vi "DSF.Shared.Configuration.Transfer.Compact Channels.vi"(11 "Channel Parameters":T2[](array[typedef]) {"Channel Ref" format="%016x"; "offset" format="%d bytes"}) -> (3 "Channel Blocks":T1[](array[typedef]) {"count" format="%d elements"; "Base Channel"."Channel Ref" format="%016x"; "Base Channel"."offset" format="%d bytes"})   [LabVIEW 2016, in "DSF.Shared.lvlib" / "DSF.Shared.Configuration.Transfer.lvclass"]
uses:
  DSF.Shared.Configuration.Transfer.lvclass
  Typedefs/DSF.Shared.Typedefs.Configuration.Transfer.Channel Parameters.ctl
  Typedefs/DSF.Shared.Typedefs.Data Type.ctl
  <vilib>/NI Veristand/Custom Device API/Custom Device Item Ref.ctl
  Typedefs/DSF.Shared.Typedefs.Configuration.Transfer.Channel Block.ctl
  DSF.Shared.lvlib
  <vilib>/NI Veristand/Custom Device API/Custom Device API.lvlib
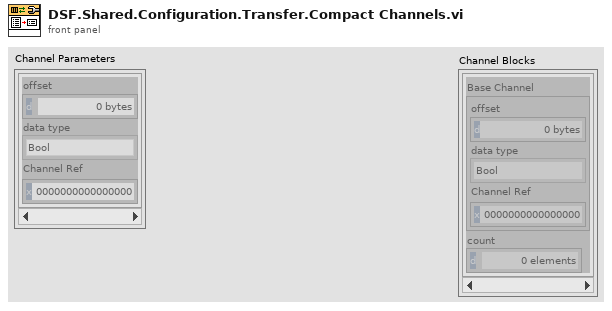
[diagram p1: front panel]
types:
  T1 = typedef "DSF.Shared.lvlib/DSF.Shared.Typedefs.Configuration.Transfer.Channel Block.ctl" = cluster{"Base Channel":T2, "count":u64}
  T2 = typedef "DSF.Shared.lvlib/DSF.Shared.Typedefs.Configuration.Transfer.Channel Parameters.ctl" = cluster{"offset":u64, "data type":T3, "Channel Ref":T4}
  T3 = typedef "DSF.Shared.lvlib/DSF.Shared.Typedefs.Data Type.ctl" = enum8{"Bool", "SGL", "DBL", "I8", "I16", "I32", "I64", "U8", "U16", "U32", "U64"}
  T4 = typedef "Custom Device API.lvlib/Custom Device Item Ref.ctl" = u64
  T5 = cluster{"offset":bool, "data type":bool, "Channel Ref":bool}
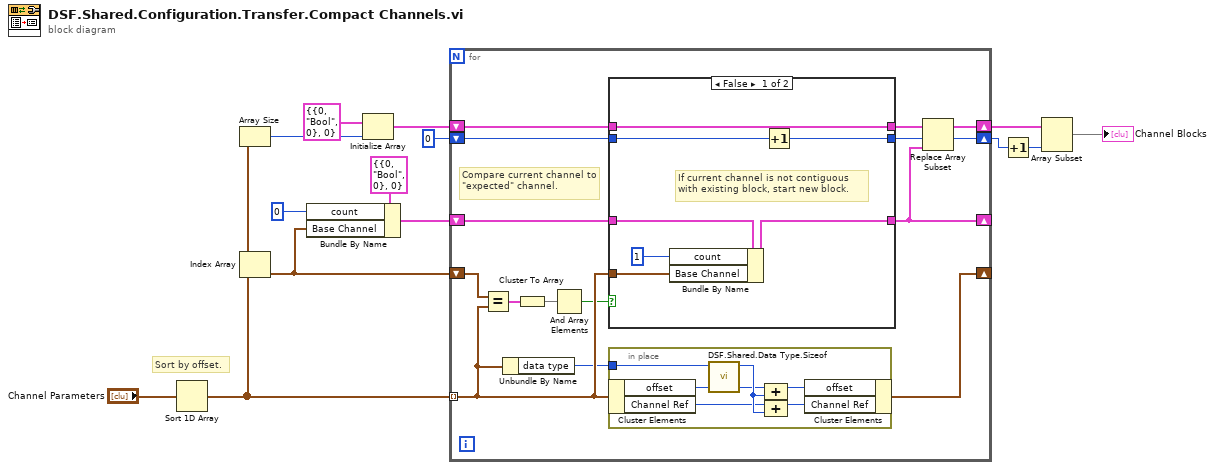
[diagram p0: block diagram]
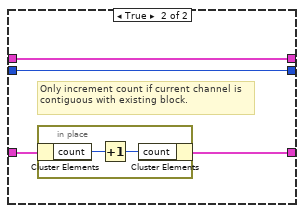
[diagram p2: hidden frame]
diagram:
  # "Sort by offset."
  n1 = Sort 1D Array(array="Channel Parameters") -> (sorted array=w6:T2[])
  n2 = Array Size(array=w6) -> (size(s)=w12:i32)
  n3 = Index Array(array=w6) -> (element=w4:T2)  [unwired: 1 in]
  n4 = Bundle By Name(cluster=T1 {"Base Channel"={"offset"=0, "data type"=enum."Bool", "Channel Ref"=0}, "count"=0} ("Channel Parameters"), "count"=u64 0, "Base Channel"=w4) -> (w3:T1)
  n5 = Initialize Array(T1 {"Base Channel"={"offset"=0, "data type"=enum."Bool", "Channel Ref"=0}, "count"=0} ("Channel Parameters"), w12) -> (w11:T1[])
  n6 = for {
    tunnel: w6 -> [w28] mode=indexing
    shift-right: [w17] -> _
    shift-left: w4 -> [w25]
    shift-right: [w20] -> w9
    shift-left: w11 -> [w23]
    shift-right: [w19] -> w8
    shift-left: 0 ("size(s)") -> [w22]
    shift-right: [w18] -> _
    shift-left: w3 -> [w24]
    # "Compare current channel to \"expected\" channel."
    n7 = Equal?(x=w25, y=w28) -> (x = y?=w27:T5)
    n8 = Unbundle By Name(w28) -> ("data type"=w16:T3)
    n9 = Cluster To Array(cluster=w27) -> (array=w26:bool[])
    n10 = And Array Elements(Boolean array=w26) -> (logical AND=w15:bool)
    n11 = case shown="False" w15 {
      tunnel: w24 -> [w39 w45]
      tunnel: [w38 w44] -> w18
      tunnel: w23 -> [w40 w43]
      tunnel: w22 -> [w41 w42]
      tunnel: [w37 w42] -> w19
      tunnel: [w40 w43] -> w21
      tunnel: w28 -> [w35 _]
      frame False {
        # "If current channel is not contiguous with existing block, start new block."
        n12 = Bundle By Name(cluster=w39, "count"=u64 1, "Base Channel"=w35) -> (w38:T1)
        n13 = Increment(x=w41) -> (x+1=w37:i32)
      }
      frame True {
        # "Only increment count if current channel is contiguous with existing block."
        n14 = in-place {
          n15 = in-place-cluster #1(w45) -> ("count"=w47:u64)
          n16 = Increment(x=w47) -> (x+1=w46:u64)
          n17 = in-place-cluster #1("count"=w46) -> (w44:T1)
        }
      }
    }
    n18 = in-place {
      in-place-border: w16 -> [w29]
      n19 = in-place-cluster #2(w28) -> ("offset"=w32:u64, "Channel Ref"=w33:T4)
      n20 = call "DSF.Shared.Data Type.Sizeof.vi"("data type"=w29) -> ("size in bytes"=w34:u64)  [unwired: 9 in, 1 out]
      n21 = Compound Arithmetic op=ADD(w32, w34) -> (w31:u64)
      n22 = Compound Arithmetic op=ADD(w33, w34) -> (w30:T4)
      n23 = in-place-cluster #2("offset"=w31, "Channel Ref"=w30) -> (w17:T2)
    }
    n24 = Replace Array Subset(array=w21, new element=w18, index=w19) -> (w20:T1[])
  }
  n25 = Increment(x=w8) -> (x+1=w1:i32)
  n26 = Array Subset(array=w9, length=w1) -> (→"Channel Blocks":T1[])  [unwired: 1 in]
